vi "Multi_LOG_4.vi"() -> ()   [LabVIEW 2014]
uses:
  <vilib>/Instr/_visa.llb/VISA Set IO Buffer Mask.ctl
  <vilib>/Instr/_visa.llb/VISA Flush IO Buffer Mask.ctl
  <vilib>/Instr/_visa.llb/VISA Configure Serial Port (Instr).vi
  picohrdl.dll
panel:
  out "Ch nr. 14":string[](array[string])
  out "Ch nr. 13":string[](array[string])
  out "Ch nr. 12":string[](array[string])
  out "Ch nr. 11":string[](array[string])
  out "Ch nr. 10":string[](array[string])
  out "Ch nr. 9":string[](array[string])
  out "Ch nr. 8":string[](array[string])
  out "Ch nr. 7":string[](array[string])
  out "Ch nr. 6":string[](array[string])
  out "Ch nr. 5":string[](array[string])
  out "Ch nr. 4":string[](array[string])
  out "Ch nr. 3":string[](array[string])
  out "Ch nr. 2.35":string[](array[string])
  out "Ch nr. 2":string[](array[string])
  out "Ch nr. 1":string[](array[string])
  out "Ch nr. 0":string[](array[string])
  out "P1 17":dbl[](graph)
  out "P1 16":dbl[](graph)
  out "P1 15":dbl[](graph)
  out "P1 14":dbl[](graph)
  out "P1 13":dbl[](graph)
  out "P1 12":dbl[](graph)
  out "P1 11":dbl[](graph)
  out "P1 10":dbl[](graph)
  out "P1 9":dbl[](graph)
  out "P1 8":dbl[](graph)
  out "P1 7":dbl[](graph)
  out "P1 6":dbl[](graph)
  out "P1 5":dbl[](graph)
  out "P1 4":dbl[](graph)
  out "P1 3":dbl[](graph)
  out "P1 2":dbl[](graph)
  in  "stop":bool
  out "noOfOpen\nChannels":i16=2
  in  "Voltage range":i32[](array[numeric])=[0, 0, 0, 0, 0, 0, 0, 0, 0, 0, 0, 0, 0, 0, 0, 0] min=0 max=6 step=1
  in  "Single ended\n(1- single)\n(0 - difer)":i32[](array[numeric])=[1, 1, 1, 1, 1, 1, 1, 1, 1, 1, 1, 1, 1, 1, 1, 1] min=0 max=1 step=1
  in  "Ch nr":bool[](array[boolean])=[FALSE, FALSE, FALSE, FALSE, FALSE, FALSE, FALSE, FALSE, FALSE, FALSE, FALSE, FALSE, FALSE, FALSE, FALSE, FALSE]
  in  "conversionTime":i16(ring)=3 items=["60 ms", "100 ms", "180 ms", "340 ms", "660 ms"]
  in  "Mains Frequency":i16(ring) items=["50 Hz", "60 Hz"]
  in  "sampleInterval_ms":i32=1000
  out "Bytes":i32(graph)=253
  in  "Save?":bool=TRUE caption="Save"
  out "Real time":timestamp=timestamp(3598016060.195616 s since 1904-01-01)
  out "Sensor3":i32[](graph)=[0, 9682, 31275, 0, 9682, 30834, 0, 9682, 31052, 0, 9682, 31052, 0, 9682, 31057, 0, 9682, 31052, 0, 9682, 31057, 0, 9682, 30834, 0, 9682, 30839, 0, 9682, 31057, 0, 9682, 30839, 0, 9682, 30839]
  out "Sensor2":i32[](graph)=[0, 21, 96, 0, 984, 877, 0, 21, 52, 0, 19, 671, 0, 913, 467, 0, 927, 660, 0, 960, 885, 0, 982, 845, 0, 987, 396, 0, 936, 541, 0, 962, 983, 0, 975, 828]
  out "Sensor1":dbl[](graph)=[0.0, 620.021, 1359.096, 0.0, 619.984, 1358.877, 0.0, 620.021, 1359.052, 0.0, 620.019, 1358.671, 0.0, 619.913, 1358.467, 0.0, 619.927, 1358.66, 0.0, 619.96, 1357.885, 0.0, 619.982, 1357.845, 0.0, 619.987, 1357.396, 0.0, 619.936, 1358.541, 0.0, 619.962, 1357.983, 0.0, 619.975, 1357.828]
  in  "VISA resource name":refnum<visa-resource-name>="COM8"
  # "1       2       3      4       5        6       7       8       9      10     11      12     13    14       15     16"
  # "0 -+2500mV\n1 -+1250mV\n2 -+625mV\n3 -+313mV\n4 -+156mV\n5 -+78mv\n6 -+39mV"
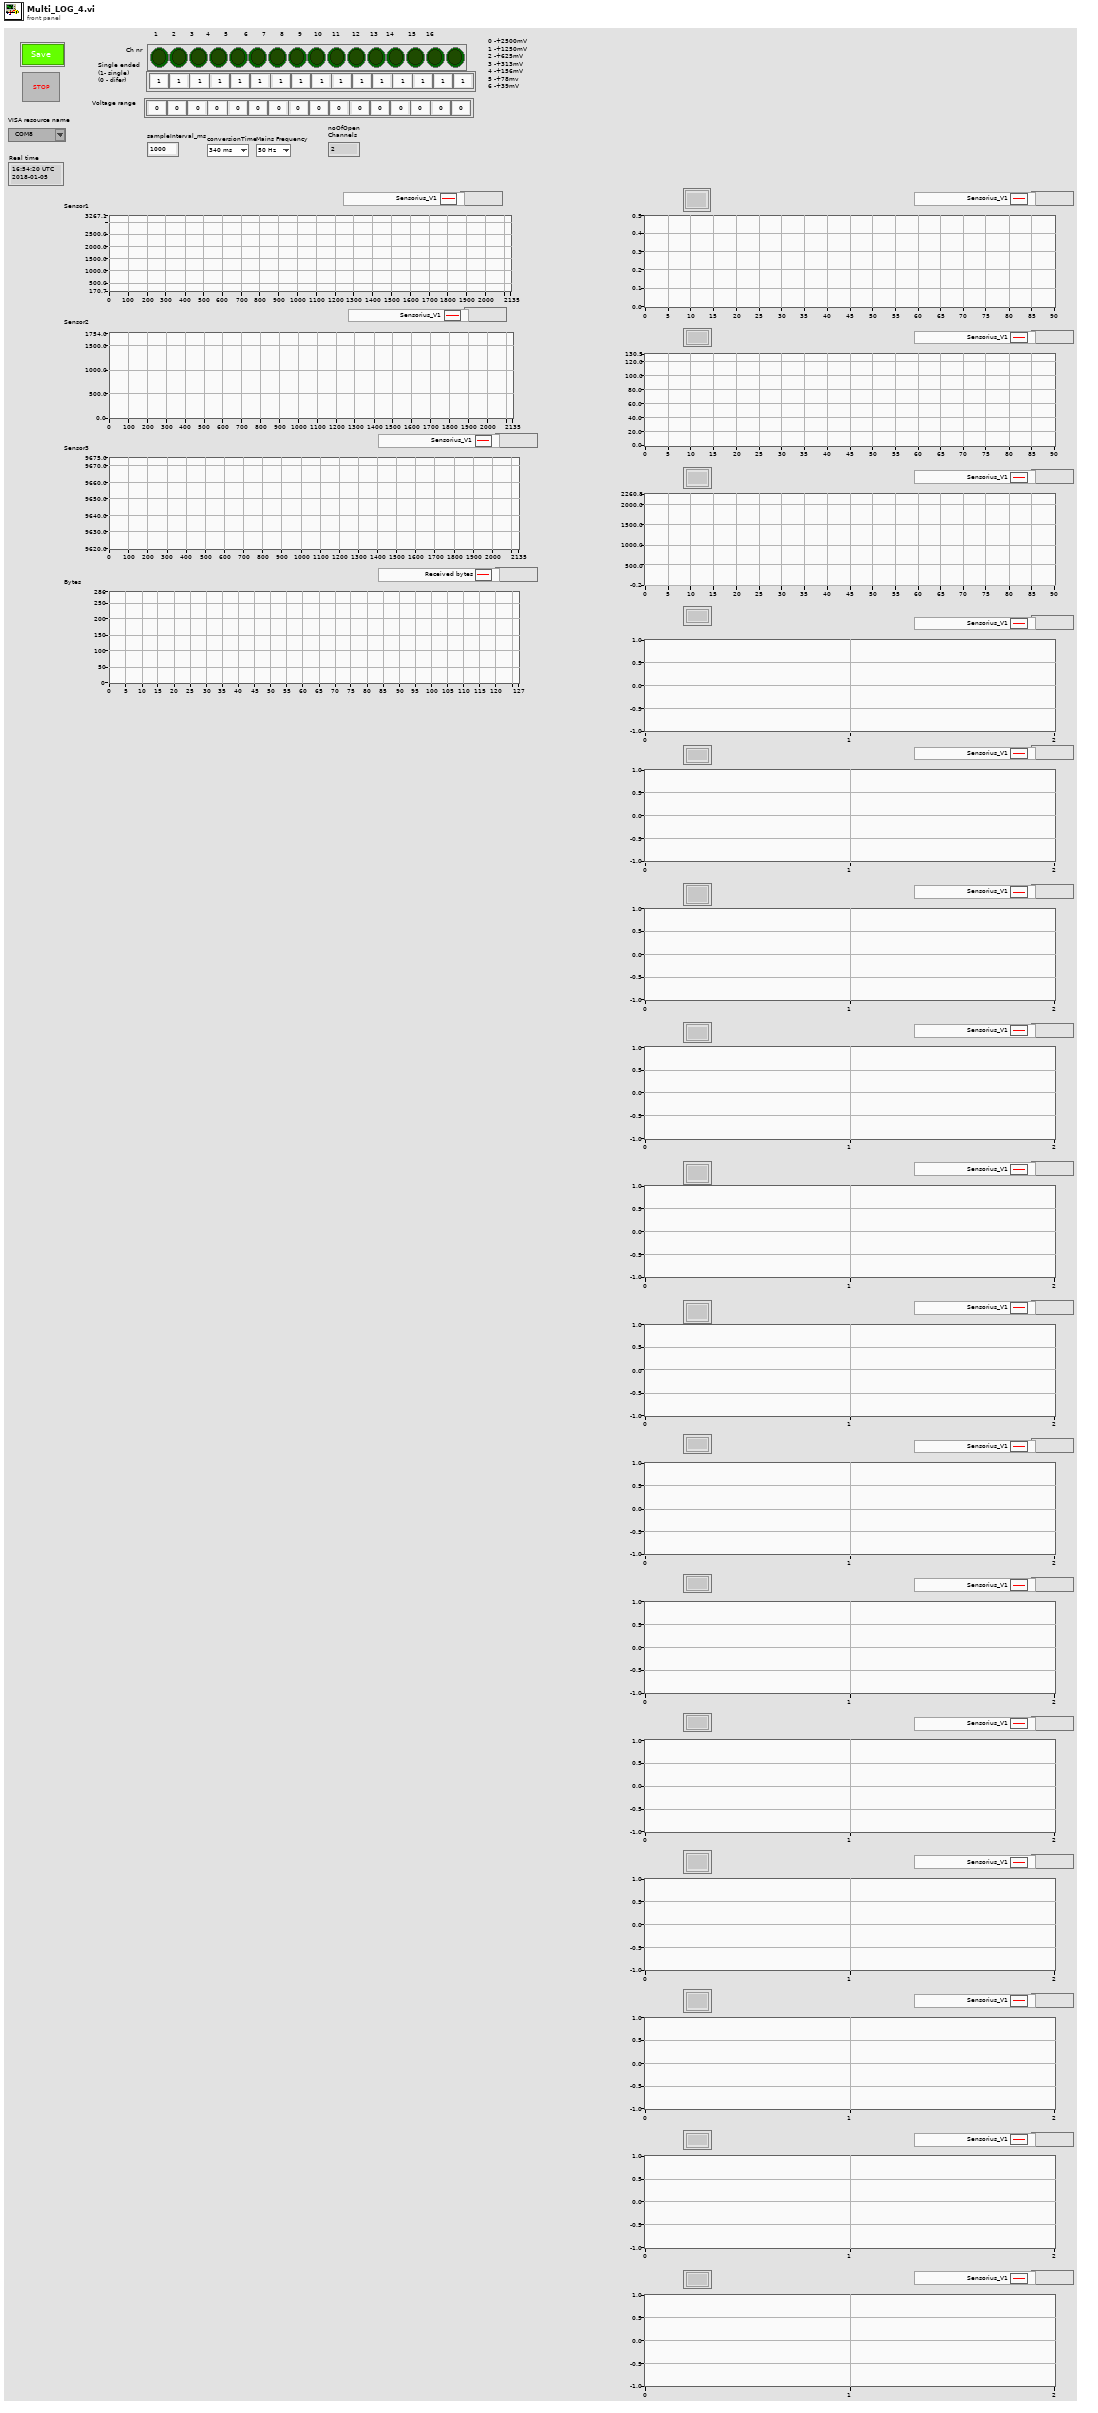
[diagram p1: front panel]
types:
  T1 = typedef "VISA Set IO Buffer Mask.ctl" = u16
  T2 = typedef "VISA Flush IO Buffer Mask.ctl" = u16
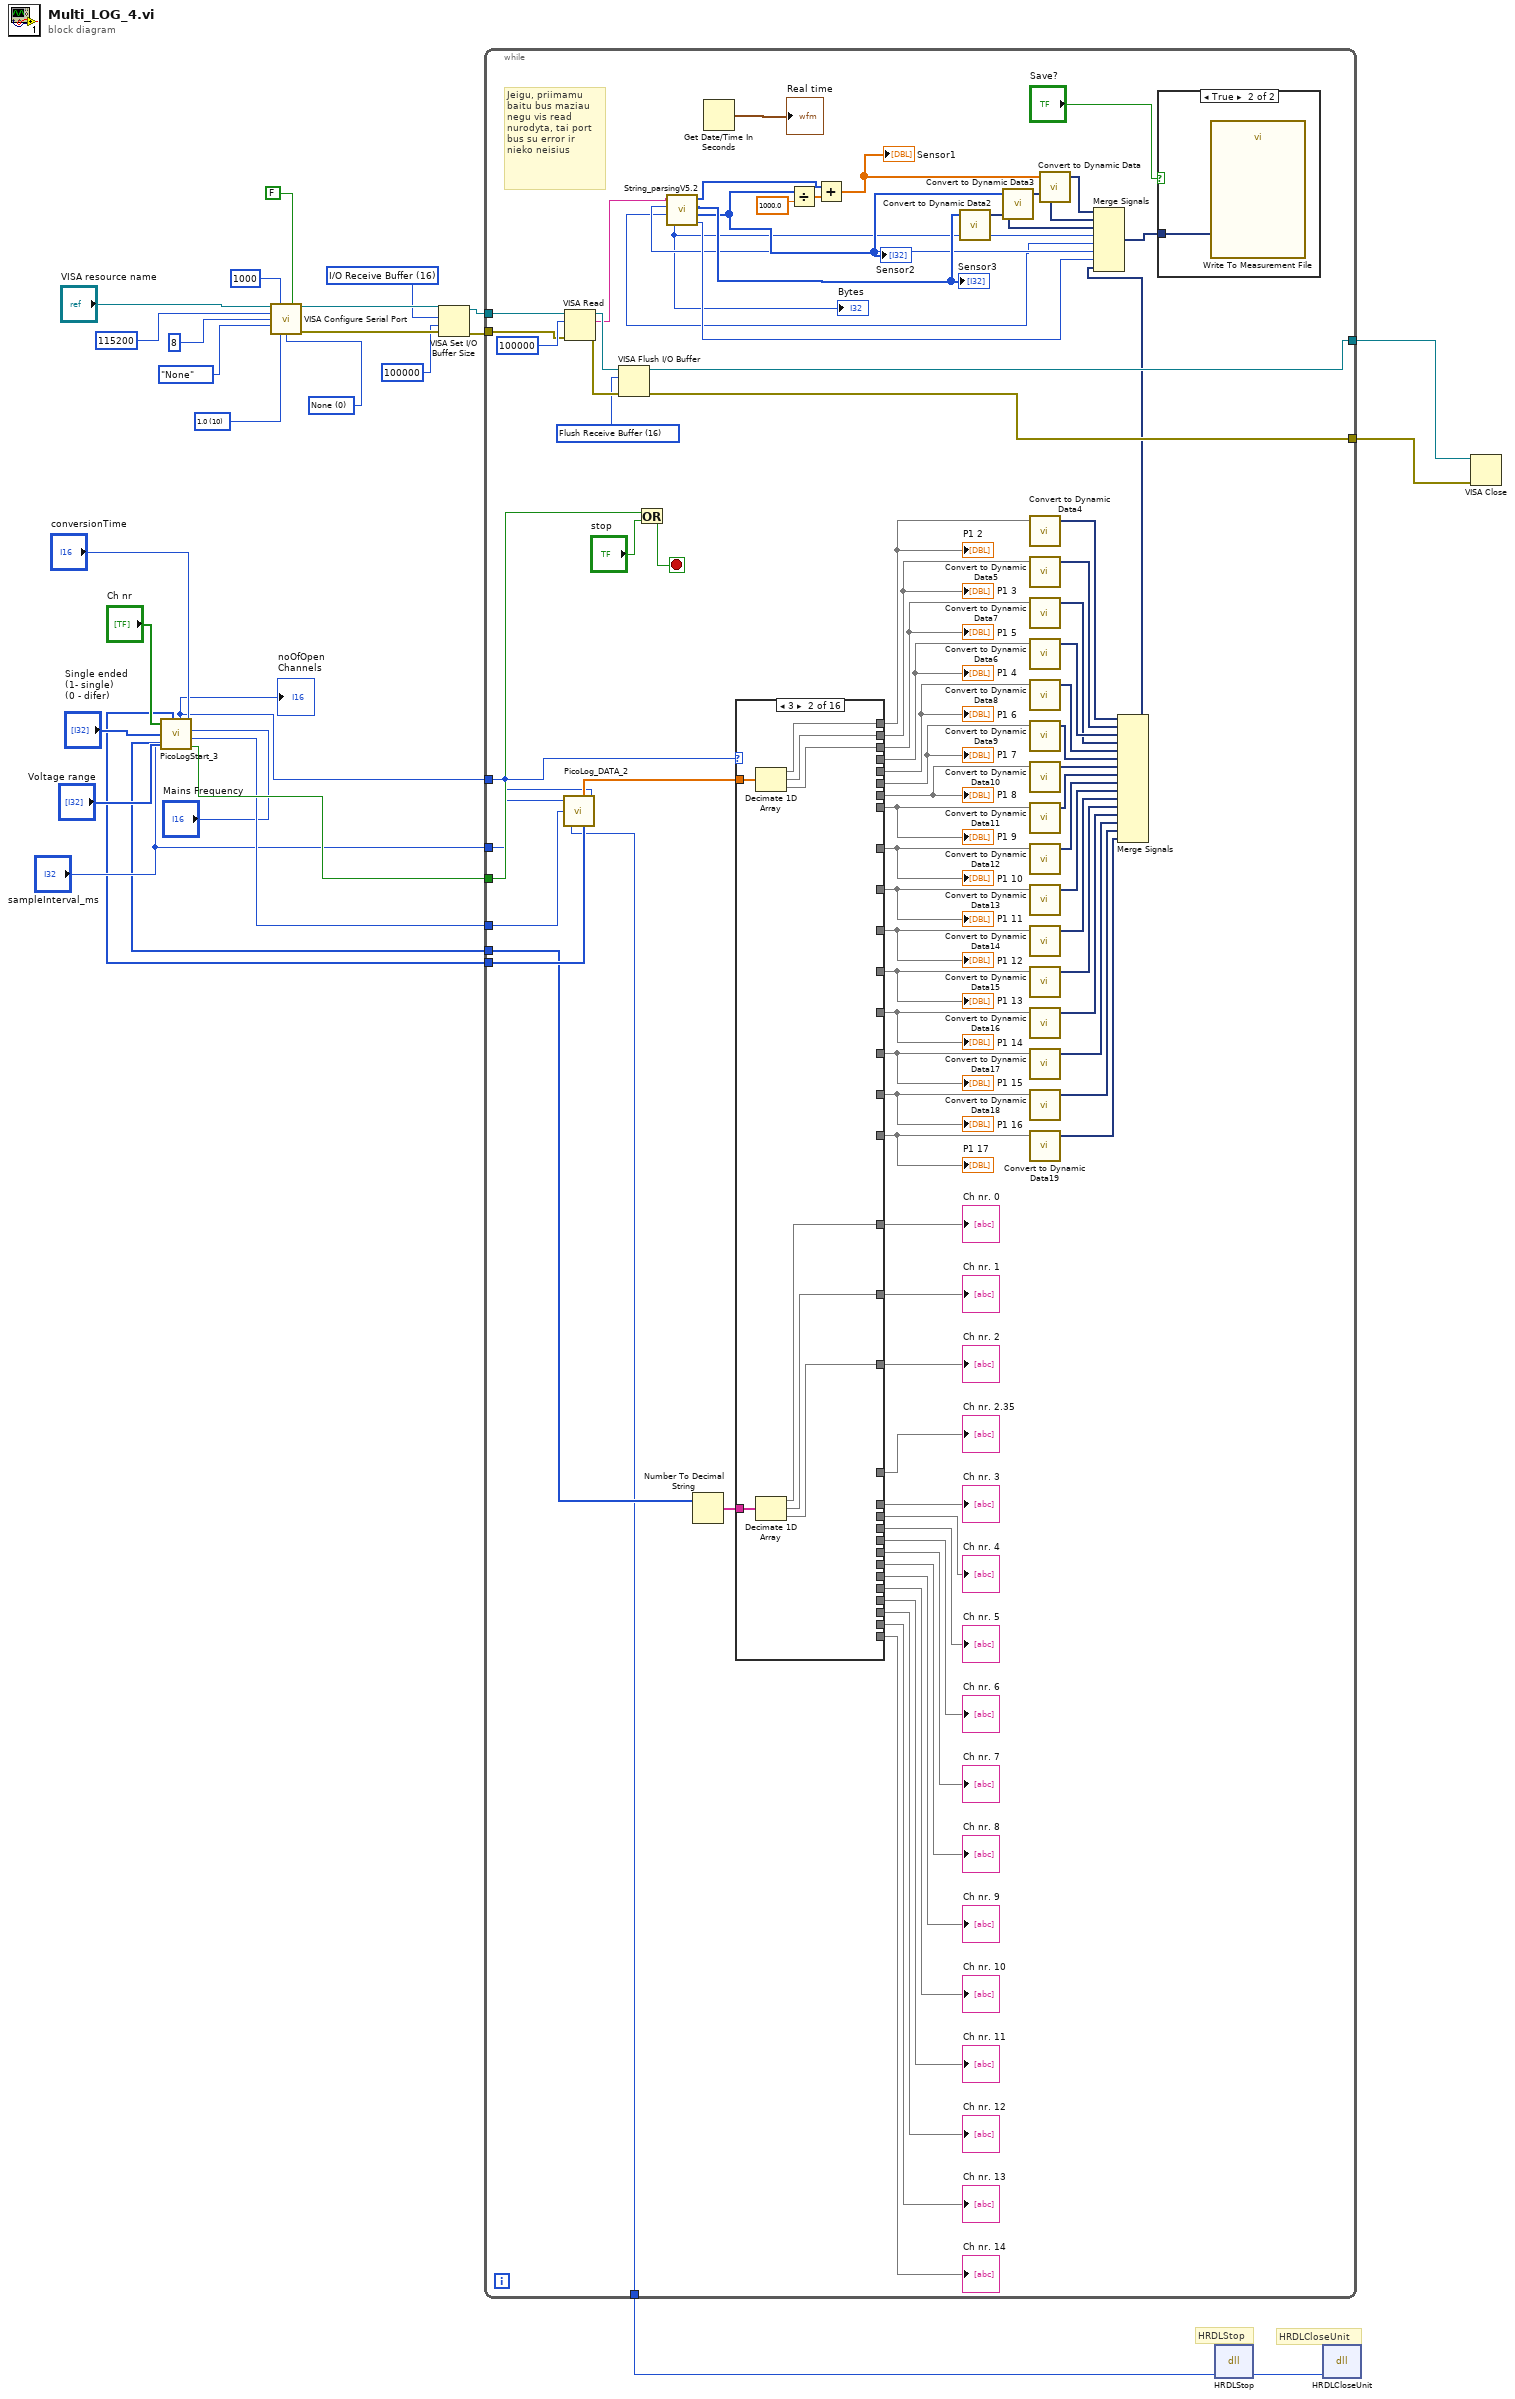
[diagram p0: block diagram]
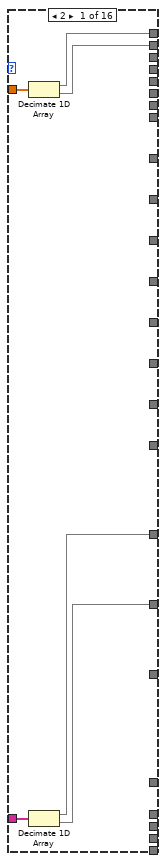
[diagram p2: hidden frame]
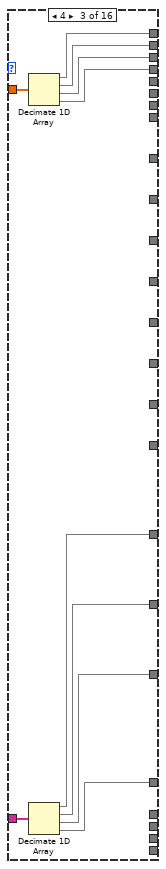
[diagram p3: hidden frame]
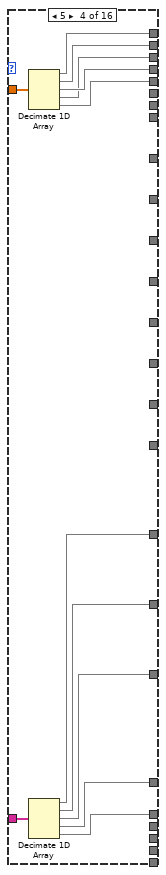
[diagram p4: hidden frame]
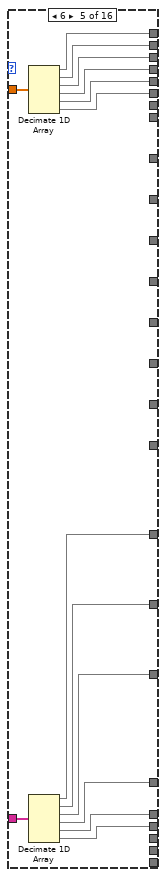
[diagram p5: hidden frame]
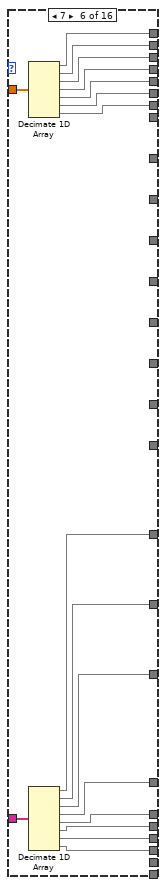
[diagram p6: hidden frame]
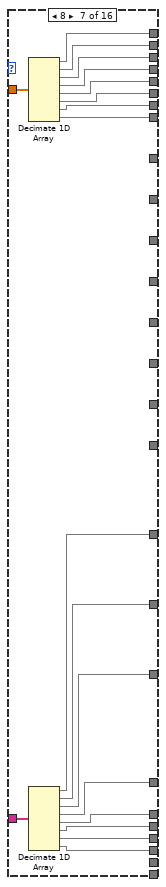
[diagram p7: hidden frame]
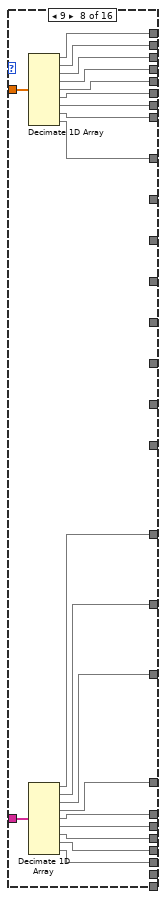
[diagram p8: hidden frame]
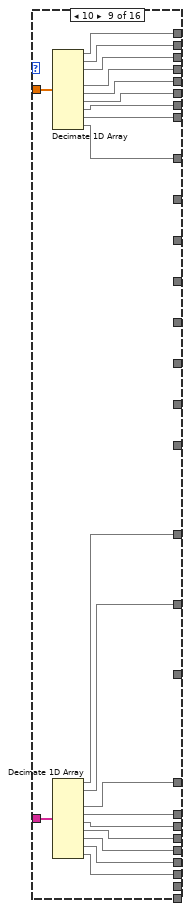
[diagram p9: hidden frame]
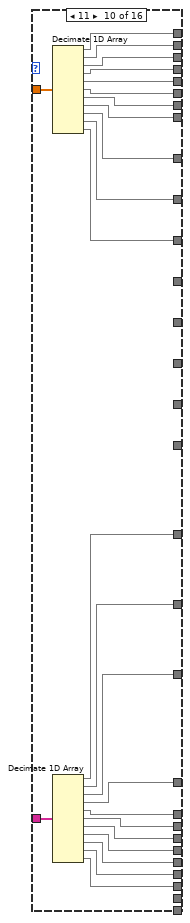
[diagram p10: hidden frame]
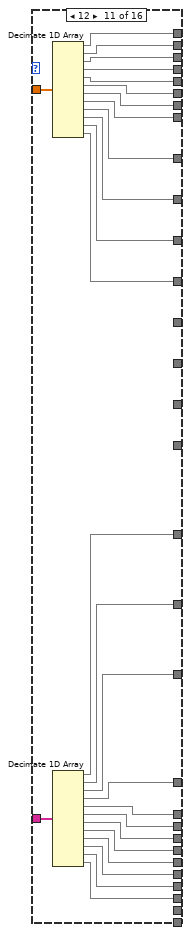
[diagram p11: hidden frame]
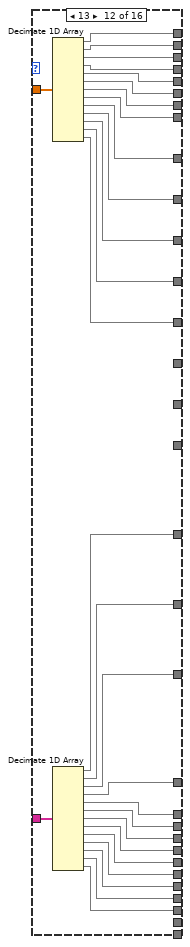
[diagram p12: hidden frame]
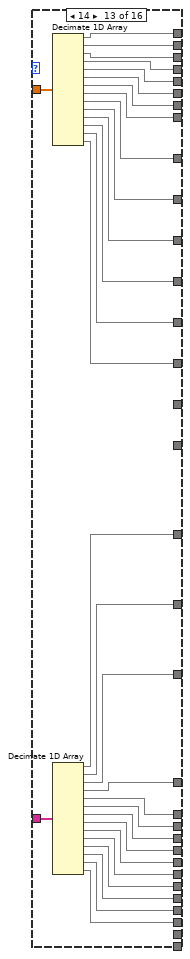
[diagram p13: hidden frame]
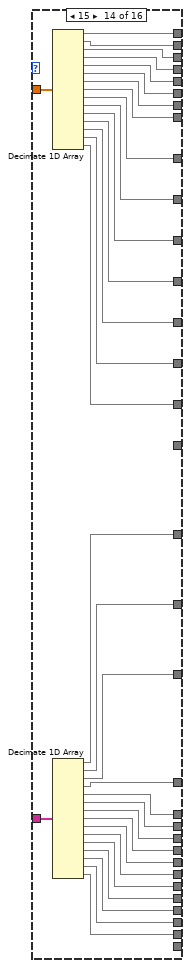
[diagram p14: hidden frame]
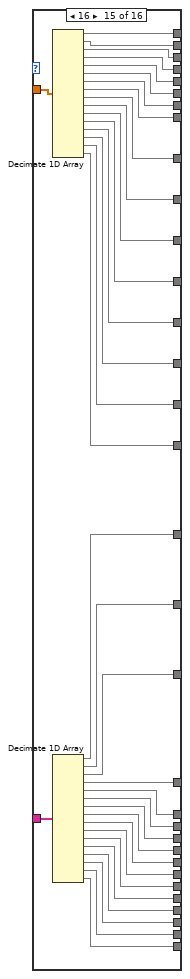
[diagram p15: hidden frame]
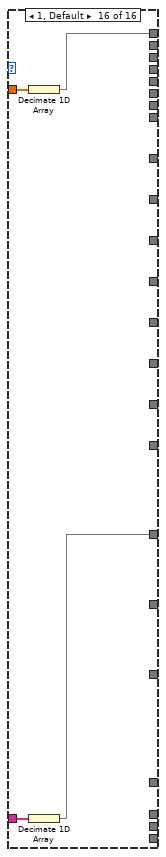
[diagram p16: hidden frame]
diagram:
  w19 = T1 16 items=["I/O Receive Buffer"=16, "I/O Transmit Buffer"=32, "I/O Receive and Transmit Buffer"=48] ("Mask")
  w25 = u16 0 items=["None", "XON/XOFF", "RTS/CTS", "XON/XOFF & RTS/CTS", "DTR/DSR", "XON/XOFF & DTR/DSR"] ("flow control (0:none)")
  w26 = u16 10 items=["1.0"=10, "1.5"=15, "2.0"=20] ("stop bits (10: 1 bit)")
  # "HRDLStop"
  # "HRDLCloseUnit"
  n1 = call "PicoLogStart_3.vi"("Ch nr"="Ch nr", "Single ended\n(0- single)\n(1 - difer)"="Single ended\n(1- single)\n(0 - difer)", "sampleInterval_ms"="sampleInterval_ms", "Voltage range"="Voltage range", "conversionTime"="conversionTime", "Mains Frequency"="Mains Frequency") -> ("Voltage range"=w1:i32[], "noOfChannels"=w7:i16, "ChNrSkArr"=w4:i32[], "handle"=w9:i16, "STOP"=w11:bool)
  "noOfOpen\nChannels" <- w7
  n2 = call-poly "VISA Configure Serial Port"("VISA resource name"="VISA resource name", "timeout (10sec)"=u32 1000, "Enable Termination\nChar (T)"=FALSE ("Enable Termination\nChar (T)"), "baud rate (9600)"=u32 115200, "data bits (8)"=u16 8, "parity (0:none)"=enum16{"None", "Odd", "Even", "Mark", "Space"}."None", "stop bits (10: 1 bit)"=w26, "flow control (0:none)"=w25) -> ("VISA resource name out"=w21:refnum<visa-resource-name>, "error out"=w22:errorcluster)  [unwired: 6 in]
  n3 = VISA Set I/O Buffer Size(VISA resource name=w21, mask (16)=w19, size (4096)=u32 100000, error in (no error)=w22) -> (VISA resource name out=w16:refnum<visa-resource-name>, error out=w18:errorcluster)
  n4 = while {
    tunnel: w16 -> [w114]
    tunnel: w18 -> [w112]
    tunnel: [w108] -> w2
    tunnel: [w107] -> w3
    tunnel: w11 -> [w36]
    tunnel: w1 -> [w38]
    tunnel: w4 -> [w37]
    tunnel: w9 -> [w35]
    tunnel: "sampleInterval_ms" -> [w34]
    tunnel: w7 -> [w33]
    tunnel: [w30] -> w5
    stop <- w32 stop-if-true
    w109 = T2 16 items=["Flush Receive Buffer"=16, "Write Transmit Buffer to Device"=32, "Flush Receive Buffer (No I/O)"=64, "Flush Transmit Buffer"=128] ("Mask")
    # "Jeigu, priimamu baitu bus maziau negu vis read nurodyta, tai port bus su error ir nieko neisius"
    n5 = call "PicoLog_DATA_2.vi"("k m"=w38, "noOfChannels"=w33, "handle"=w35, "sampleInterval_ms"=w34) -> ("x*y"=w71:dbl[], "handle"=w30:i16)  [unwired: 3 in]
    n6 = VISA Read(VISA resource name=w114, byte count=u32 100000, error in (no error)=w112) -> (VISA resource name out=w111:refnum<visa-resource-name>, read buffer=w98:string, error out=w110:errorcluster)  [unwired: 1 out]
    n7 = VISA Flush I/O Buffer(VISA resource name=w111, mask (16)=w109, error in (no error)=w110) -> (VISA resource name out=w108:refnum<visa-resource-name>, error out=w107:errorcluster)
    n8 = Or(x=w36, y="stop") -> (x .or. y?=w32:bool)
    n9 = call "String_parsingV5.2.vi"("input string"=w98) -> ("hour"=w97:i32, "V2"=w94:i32[], "V3"=w95:i32[], "V1"=w96:i32[], "size(s)"=w90:i32, "sekundes"=w92:i32, "minute"=w93:i32)
    "Sensor2" <- w94
    "Sensor3" <- w95
    "Bytes" <- w90
    n10 = Number To Decimal String(number=w37) -> (decimal integer string=w87:string[])  [unwired: 1 in]
    n11 = Get Date/Time In Seconds() -> (seconds since 1Jan1904=→"Real time":timestamp)
    n12 = case shown="3" w33 {
      tunnel: w71 -> [w120 w128 w138 w150 w164 w181 w199 w219 w239 w263 w289 w317 w347 w379 w413 w417]
      tunnel: [w119 w127 w137 w149 w163 w180 w198 w218 w238 w262 w288 w316 w346 w378 w412 w416] -> w70
      tunnel: [w118 w126 w136 w148 w162 w179 w197 w217 w237 w261 w287 w315 w345 w377 w411 _] -> w68
      tunnel: [_ _ w134 w147 w160 w177 w195 w215 w235 w260 w285 w313 w343 w375 w409 _] -> w66
      tunnel: [_ w125 w135 w146 w161 w178 w196 w216 w236 w259 w286 w314 w344 w376 w410 _] -> w64
      tunnel: [_ _ _ w145 w159 w176 w194 w214 w234 w258 w284 w312 w342 w374 w408 _] -> w62
      tunnel: [_ _ _ _ w158 w175 w193 w213 w233 w257 w283 w311 w341 w373 w407 _] -> w60
      tunnel: [_ _ _ _ _ w174 w192 w212 w232 w256 w282 w310 w340 w372 w406 _] -> w58
      tunnel: [_ _ _ _ _ _ w191 w211 w231 w255 w281 w309 w339 w371 w405 _] -> w56
      tunnel: [_ _ _ _ _ _ _ w210 w230 w254 w280 w308 w338 w370 w404 _] -> w54
      tunnel: [_ _ _ _ _ _ _ _ _ w253 w279 w307 w337 w369 w403 _] -> w52
      tunnel: [_ _ _ _ _ _ _ _ _ w252 w278 w306 w336 w368 w402 _] -> w50
      tunnel: [_ _ _ _ _ _ _ _ _ _ w277 w305 w335 w367 w401 _] -> w48
      tunnel: [_ _ _ _ _ _ _ _ _ _ _ w304 w334 w366 w400 _] -> w46
      tunnel: [_ _ _ _ _ _ _ _ _ _ _ _ w333 w365 w399 _] -> w44
      tunnel: [_ _ _ _ _ _ _ _ _ _ _ _ _ w364 w398 _] -> w42
      tunnel: [_ _ _ _ _ _ _ _ _ _ _ _ _ _ w397 _] -> w40
      tunnel: [_ _ _ _ _ _ _ _ _ _ _ _ _ _ w396 _] -> w88
      tunnel: w87 -> [w117 w124 w133 w144 w157 w173 w190 w209 w229 w251 w276 w303 w332 w363 w395 w415]
      tunnel: [w116 w123 w132 w143 w156 w172 w189 w208 w228 w250 w275 w302 w331 w362 w394 w414] -> w86
      tunnel: [_ _ _ _ _ _ _ _ _ _ _ _ _ w348 w380 _] -> w85
      tunnel: [w115 w122 w131 w142 w155 w171 w188 w207 w227 w249 w274 w301 w330 w361 w393 _] -> w84
      tunnel: [_ w121 w130 w141 w154 w170 w187 w206 _ w248 w273 w300 w329 w360 w392 _] -> w83
      tunnel: [_ _ w129 w140 w153 w169 w186 w205 w226 w247 w272 w299 w328 w359 w391 _] -> w82
      tunnel: [_ _ _ w139 w152 w168 w185 w204 w225 w246 w271 w298 w327 w358 w390 _] -> w72
      tunnel: [_ _ _ _ w151 w167 w184 w203 w224 w245 w270 w297 w326 w357 w389 _] -> w81
      tunnel: [_ _ _ _ _ w166 w183 w202 w223 w244 w269 w296 w325 w356 w388 _] -> w80
      tunnel: [_ _ _ _ _ w165 w182 w201 w222 w243 w268 w295 w324 w355 w387 _] -> w79
      tunnel: [_ _ _ _ _ _ _ w200 w221 w242 w267 w294 w323 w354 w386 _] -> w78
      tunnel: [_ _ _ _ _ _ _ _ w220 w241 w266 w293 w322 w353 w385 _] -> w77
      tunnel: [_ _ _ _ _ _ _ _ _ w240 w265 w292 w321 w352 w384 _] -> w76
      tunnel: [_ _ _ _ _ _ _ _ _ _ w264 w291 w320 w351 w383 _] -> w75
      tunnel: [_ _ _ _ _ _ _ _ _ _ _ w290 w319 w350 w382 _] -> w74
      tunnel: [_ _ _ _ _ _ _ _ _ _ _ _ w318 w349 w381 _] -> w73
      frame 2 {
        n13 = Decimate 1D Array(w120) -> (w119:dbl[], w118:dbl[])
        n14 = Decimate 1D Array(w117) -> (w116:string[], w115:string[])
      }
      frame 3 {
        n15 = Decimate 1D Array(w128) -> (w127:dbl[], w126:dbl[], w125:dbl[])
        n16 = Decimate 1D Array(w124) -> (w123:string[], w122:string[], w121:string[])
      }
      frame 4 {
        n17 = Decimate 1D Array(w138) -> (w137:dbl[], w136:dbl[], w135:dbl[], w134:dbl[])
        n18 = Decimate 1D Array(w133) -> (w132:string[], w131:string[], w130:string[], w129:string[])
      }
      frame 5 {
        n19 = Decimate 1D Array(w150) -> (w149:dbl[], w148:dbl[], w147:dbl[], w146:dbl[], w145:dbl[])
        n20 = Decimate 1D Array(w144) -> (w143:string[], w142:string[], w141:string[], w140:string[], w139:string[])
      }
      frame 6 {
        n21 = Decimate 1D Array(w164) -> (w163:dbl[], w162:dbl[], w161:dbl[], w160:dbl[], w159:dbl[], w158:dbl[])
        n22 = Decimate 1D Array(w157) -> (w156:string[], w155:string[], w154:string[], w153:string[], w152:string[], w151:string[])
      }
      frame 7 {
        n23 = Decimate 1D Array(w181) -> (w180:dbl[], w179:dbl[], w178:dbl[], w177:dbl[], w176:dbl[], w175:dbl[], w174:dbl[])
        n24 = Decimate 1D Array(w173) -> (w172:string[], w171:string[], w170:string[], w169:string[], w168:string[], w167:string[], w166:string[], w165:string[])
      }
      frame 8 {
        n25 = Decimate 1D Array(w199) -> (w198:dbl[], w197:dbl[], w196:dbl[], w195:dbl[], w194:dbl[], w193:dbl[], w192:dbl[], w191:dbl[])
        n26 = Decimate 1D Array(w190) -> (w189:string[], w188:string[], w187:string[], w186:string[], w185:string[], w184:string[], w183:string[], w182:string[])
      }
      frame 9 {
        n27 = Decimate 1D Array(w219) -> (w218:dbl[], w217:dbl[], w216:dbl[], w215:dbl[], w214:dbl[], w213:dbl[], w212:dbl[], w211:dbl[], w210:dbl[])
        n28 = Decimate 1D Array(w209) -> (w208:string[], w207:string[], w206:string[], w205:string[], w204:string[], w203:string[], w202:string[], w201:string[], w200:string[])
      }
      frame 10 {
        n29 = Decimate 1D Array(w239) -> (w238:dbl[], w237:dbl[], w236:dbl[], w235:dbl[], w234:dbl[], w233:dbl[], w232:dbl[], w231:dbl[], w230:dbl[])  [unwired: 1 out]
        n30 = Decimate 1D Array(w229) -> (w228:string[], w227:string[], w226:string[], w225:string[], w224:string[], w223:string[], w222:string[], w221:string[], w220:string[])  [unwired: 1 out]
      }
      frame 11 {
        n31 = Decimate 1D Array(w263) -> (w262:dbl[], w261:dbl[], w259:dbl[], w260:dbl[], w258:dbl[], w257:dbl[], w256:dbl[], w255:dbl[], w254:dbl[], w253:dbl[], w252:dbl[])
        n32 = Decimate 1D Array(w251) -> (w250:string[], w249:string[], w248:string[], w247:string[], w246:string[], w245:string[], w244:string[], w243:string[], w242:string[], w241:string[], w240:string[])
      }
      frame 12 {
        n33 = Decimate 1D Array(w289) -> (w288:dbl[], w287:dbl[], w286:dbl[], w285:dbl[], w284:dbl[], w283:dbl[], w282:dbl[], w281:dbl[], w280:dbl[], w279:dbl[], w278:dbl[], w277:dbl[])
        n34 = Decimate 1D Array(w276) -> (w275:string[], w274:string[], w273:string[], w272:string[], w271:string[], w270:string[], w269:string[], w268:string[], w267:string[], w266:string[], w265:string[], w264:string[])
      }
      frame 13 {
        n35 = Decimate 1D Array(w317) -> (w316:dbl[], w315:dbl[], w314:dbl[], w313:dbl[], w312:dbl[], w311:dbl[], w310:dbl[], w309:dbl[], w308:dbl[], w307:dbl[], w306:dbl[], w305:dbl[], w304:dbl[])
        n36 = Decimate 1D Array(w303) -> (w302:string[], w301:string[], w300:string[], w299:string[], w298:string[], w297:string[], w296:string[], w295:string[], w294:string[], w293:string[], w292:string[], w291:string[], w290:string[])
      }
      frame 14 {
        n37 = Decimate 1D Array(w347) -> (w346:dbl[], w345:dbl[], w344:dbl[], w343:dbl[], w342:dbl[], w341:dbl[], w340:dbl[], w339:dbl[], w338:dbl[], w337:dbl[], w336:dbl[], w335:dbl[], w334:dbl[], w333:dbl[])
        n38 = Decimate 1D Array(w332) -> (w331:string[], w330:string[], w329:string[], w328:string[], w327:string[], w326:string[], w325:string[], w324:string[], w323:string[], w322:string[], w321:string[], w320:string[], w319:string[], w318:string[])
      }
      frame 15 {
        n39 = Decimate 1D Array(w379) -> (w378:dbl[], w377:dbl[], w376:dbl[], w375:dbl[], w374:dbl[], w373:dbl[], w372:dbl[], w371:dbl[], w370:dbl[], w369:dbl[], w368:dbl[], w367:dbl[], w366:dbl[], w365:dbl[], w364:dbl[])
        n40 = Decimate 1D Array(w363) -> (w362:string[], w361:string[], w360:string[], w359:string[], w358:string[], w357:string[], w356:string[], w355:string[], w354:string[], w353:string[], w352:string[], w351:string[], w350:string[], w349:string[], w348:string[])
      }
      frame 16 {
        n41 = Decimate 1D Array(w413) -> (w412:dbl[], w411:dbl[], w410:dbl[], w409:dbl[], w408:dbl[], w407:dbl[], w406:dbl[], w405:dbl[], w404:dbl[], w403:dbl[], w402:dbl[], w401:dbl[], w400:dbl[], w399:dbl[], w398:dbl[], w397:dbl[])
        n42 = Decimate 1D Array(w395) -> (w394:string[], w393:string[], w392:string[], w391:string[], w390:string[], w389:string[], w388:string[], w387:string[], w386:string[], w385:string[], w384:string[], w383:string[], w382:string[], w381:string[], w380:string[], w396:string[])
      }
      frame 1, Default {
        n43 = Decimate 1D Array(w417) -> (w416:dbl[])
        n44 = Decimate 1D Array(w415) -> (w414:string[])
      }
    }
    "P1 2" <- w70
    "P1 3" <- w68
    "P1 4" <- w66
    "P1 5" <- w64
    "P1 6" <- w62
    "P1 7" <- w60
    "P1 8" <- w58
    "P1 9" <- w56
    "P1 10" <- w54
    "P1 11" <- w52
    "P1 12" <- w50
    "P1 13" <- w48
    "P1 14" <- w46
    "P1 15" <- w44
    "P1 16" <- w42
    "P1 17" <- w40
    "Ch nr. 0" <- w86
    "Ch nr. 1" <- w84
    "Ch nr. 2" <- w83
    "Ch nr. 2.35" <- w82
    "Ch nr. 3" <- w72
    "Ch nr. 4" <- w81
    "Ch nr. 5" <- w80
    "Ch nr. 6" <- w79
    "Ch nr. 7" <- w78
    "Ch nr. 8" <- w77
    "Ch nr. 9" <- w76
    "Ch nr. 10" <- w75
    "Ch nr. 11" <- w74
    "Ch nr. 12" <- w73
    "Ch nr. 13" <- w85
    "Ch nr. 14" <- w88
    n45 = Divide(x=w94, y=1000.0) -> (x/y=w102:dbl[])
    n46 = Add(x=w96, y=w102) -> (x+y=w100:dbl[])
    "Sensor1" <- w100
    n47 = call "Convert to Dynamic Data2"("Array"=w95) -> ("Dynamic Data Type"=w105:dynamicdata)  [unwired: 3 in]
    n48 = call "Convert to Dynamic Data3"("Array"=w94) -> ("Dynamic Data Type"=w104:dynamicdata)  [unwired: 3 in]
    n49 = call "Convert to Dynamic Data4"("Array"=w70) -> ("Dynamic Data Type"=w69:dynamicdata)  [unwired: 3 in]
    n50 = call "Convert to Dynamic Data5"("Array"=w68) -> ("Dynamic Data Type"=w67:dynamicdata)  [unwired: 3 in]
    n51 = call "Convert to Dynamic Data7"("Array"=w64) -> ("Dynamic Data Type"=w63:dynamicdata)  [unwired: 3 in]
    n52 = call "Convert to Dynamic Data6"("Array"=w66) -> ("Dynamic Data Type"=w65:dynamicdata)  [unwired: 3 in]
    n53 = call "Convert to Dynamic Data8"("Array"=w62) -> ("Dynamic Data Type"=w61:dynamicdata)  [unwired: 3 in]
    n54 = call "Convert to Dynamic Data9"("Array"=w60) -> ("Dynamic Data Type"=w59:dynamicdata)  [unwired: 3 in]
    n55 = call "Convert to Dynamic Data10"("Array"=w58) -> ("Dynamic Data Type"=w57:dynamicdata)  [unwired: 3 in]
    n56 = call "Convert to Dynamic Data11"("Array"=w56) -> ("Dynamic Data Type"=w55:dynamicdata)  [unwired: 3 in]
    n57 = call "Convert to Dynamic Data12"("Array"=w54) -> ("Dynamic Data Type"=w53:dynamicdata)  [unwired: 3 in]
    n58 = call "Convert to Dynamic Data13"("Array"=w52) -> ("Dynamic Data Type"=w51:dynamicdata)  [unwired: 3 in]
    n59 = call "Convert to Dynamic Data14"("Array"=w50) -> ("Dynamic Data Type"=w49:dynamicdata)  [unwired: 3 in]
    n60 = call "Convert to Dynamic Data15"("Array"=w48) -> ("Dynamic Data Type"=w47:dynamicdata)  [unwired: 3 in]
    n61 = call "Convert to Dynamic Data16"("Array"=w46) -> ("Dynamic Data Type"=w45:dynamicdata)  [unwired: 3 in]
    n62 = call "Convert to Dynamic Data17"("Array"=w44) -> ("Dynamic Data Type"=w43:dynamicdata)  [unwired: 3 in]
    n63 = call "Convert to Dynamic Data18"("Array"=w42) -> ("Dynamic Data Type"=w41:dynamicdata)  [unwired: 3 in]
    n64 = call "Convert to Dynamic Data19"("Array"=w40) -> ("Dynamic Data Type"=w39:dynamicdata)  [unwired: 3 in]
    n65 = call "Convert to Dynamic Data"("Array"=w100) -> ("Dynamic Data Type"=w106:dynamicdata)  [unwired: 3 in]
    n66 = Merge Signals(w69, w67, w65, w63, w61, w59, w57, w55, w53, w51, w49, w47, w45, w43, w41, w39) -> (w31:dynamicdata)
    n67 = Merge Signals(w106, w104, w105, w90, w92, w93, w97, w31) -> (w99:dynamicdata)
    n68 = case shown="True" "Save?" {
      tunnel: w99 -> [_ w418]
      frame False {
      }
      frame True {
        n69 = call "Write To Measurement File"("Signals"=w418) -> ()  [unwired: 16 in, 3 out]
      }
    }
  }
  n70 = dll-call lib="picohrdl.dll" fn="HRDLStop"("handle"=w5) -> ("handle"=w15:i16)  [unwired: 4 in, 2 out]
  n71 = dll-call lib="PicoHRDL.dll" fn="HRDLCloseUnit"("handle"=w15) -> ()  [unwired: 5 in, 2 out]
  n72 = VISA Close(VISA resource name=w2, error in (no error)=w3) -> ()  [unwired: 1 out]
